vi "寻找最高线（0黑线）.vi"(1 "允许偏差（0-100）":i32, 2 "初始位置":i32, 3 "Image":T1) -> (0 "Y位置":i32)   [LabVIEW 2017]
uses:
  <vilib>/vision/Image Controls.llb/IMAQ Image.ctl
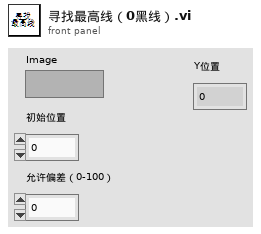
[diagram p1: front panel]
types:
  T1 = typedef "IMAQ Image.ctl" = refnum<image>
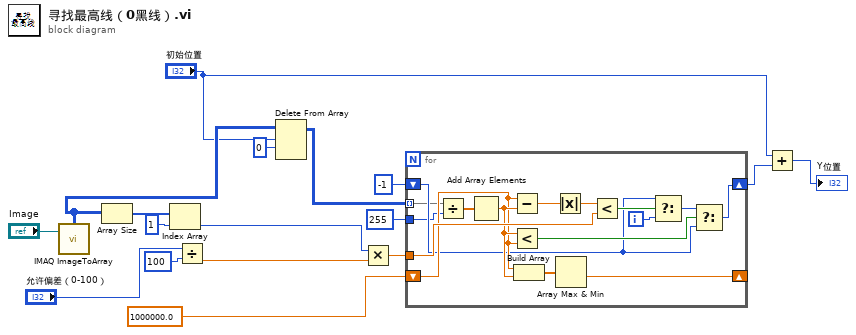
[diagram p0: block diagram]
diagram:
  n1 = call "IMAQ ImageToArray"("Image"="Image") -> ("Image Pixels (U8)"=w6:u8[][])  [unwired: 3 in, 4 out]
  n2 = Array Size(array=w6) -> (size(s)=w15:i32[])
  n3 = Index Array(array=w15, index=1 ("索引")) -> (element=w11:i32)
  n4 = Divide(x="允许偏差（0-100）", y=100) -> (x/y=w8:dbl)
  n5 = Delete From Array(array=w6, length="初始位置", index (row)=0 ("索引 (行)")) -> (array with subset deleted=w4:u8[][])  [unwired: 1 in, 1 out]
  n6 = Multiply(x=w11, y=w8) -> (x*y=w10:dbl)
  n7 = for {
    tunnel: w4 -> [w20] mode=indexing
    shift-right: [w28] -> _
    shift-left: 1000000.0 -> [w26]
    tunnel: w10 -> [w31]
    shift-right: [w21] -> w2
    shift-left: -1 -> [w22]
    tunnel: 255 ("y") -> [w19]
    i -> [w24]
    n8 = Divide(x=w20, y=w19) -> (x/y=w18:dbl[])
    n9 = Add Array Elements(numeric array=w18) -> (sum=w27:dbl)
    n10 = Subtract(x=w26, y=w27) -> (x-y=w33:dbl)
    n11 = Less?(x=w27, y=w26) -> (x < y?=w25:bool)
    n12 = Build Array(w26, w27) -> (w29:dbl[])
    n13 = Absolute Value(x=w33) -> (abs(x)=w32:dbl)
    n14 = Array Max & Min(array=w29) -> (min value=w28:dbl)  [unwired: 3 out]
    n15 = Less?(x=w32, y=w31) -> (x < y?=w30:bool)
    n16 = Select(t=w22, s=w30, f=w24) -> (s? t:f=w23:i32)
    n17 = Select(t=w23, s=w25, f=w22) -> (s? t:f=w21:i32)
  }
  n18 = Add(x="初始位置", y=w2) -> (x+y=→"Y位置":i32)
